vi "FilterChannels.vi"(8 "error in (no error)":errorcluster, 10 "Property":string, 11 "Specified Channel Ref List":T1[](array[typedef]) format="%.0x") -> (0 "error out":errorcluster, 3 "Filtered Channel list":T1[](array[typedef]) format="%.0x")   [LabVIEW 2020, in "Shared Variables CD 2.0 Engine.lvlib"]
doc: "Row 1: DBL\nRow 2 Bool"
uses:
  Shared Variables CD 2.0 Engine.lvlib
  <vilib>/NI VeriStand/Custom Device API/Custom Device Item Ref.ctl
  <vilib>/Utility/VariantDataType/Type.ctl
  <vilib>/Utility/VariantDataType/VariantType.lvlib
  <vilib>/NI VeriStand/Custom Device API/Custom Device API.lvlib
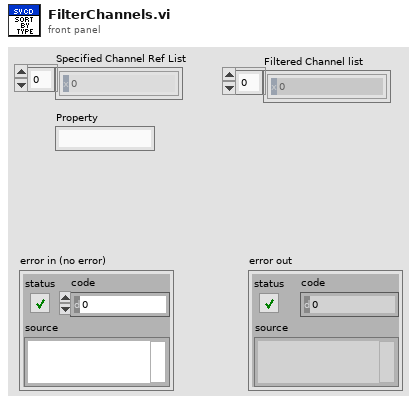
[diagram p1: front panel]
types:
  T1 = typedef "Custom Device API.lvlib/Custom Device Item Ref.ctl" = u64
  T2 = typedef "VariantType.lvlib/Type.ctl" = enum8{"Invalid Type", "Void", "I8", "I16", "I32", "I64", "U8", "U16", "U32", "U64", "Single Float", "Double Float", "Extended Float", "Single Complex", "Double Complex", "Extended Complex", "Enum U8", "Enum U16", "Enum U32", "Enum U64", "Single Float With Unit", "Double Float With Unit", "Extended Float With Unit", "Single Complex with Unit", "Double Complex with Unit", "Extended Complex with Unit", "Boolean", "String", "Path", "Picture", "Tag", "Array", "Cluster", "Variant", "LV Variant", "Waveform", "Timestamp", "Digital Waveform", "Digital Data", "ExpressData", "Refnum", "External Data", "VI", "Poly VI", "LabVIEW Class Instance", "Fixed Point"}
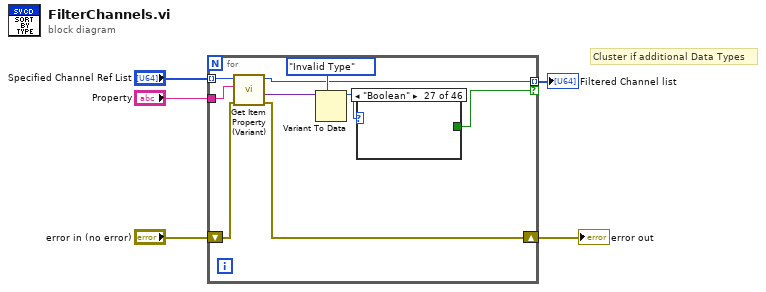
[diagram p0: block diagram]
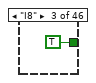
[diagram p4: hidden frame]
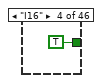
[diagram p5: hidden frame]
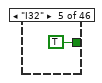
[diagram p6: hidden frame]
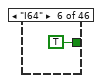
[diagram p7: hidden frame]
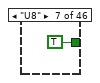
[diagram p8: hidden frame]
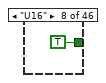
[diagram p9: hidden frame]
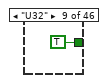
[diagram p10: hidden frame]
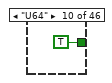
[diagram p11: hidden frame]
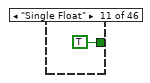
[diagram p12: hidden frame]
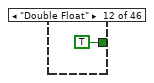
[diagram p13: hidden frame]
diagram:
  # "Cluster if additional Data Types"
  n1 = for {
    tunnel: "Specified Channel Ref List" -> [w10] mode=indexing
    tunnel: "Property" -> [w14]
    shift-right: [w8] -> w2
    shift-left: "error in (no error)" -> [w9]
    tunnel: [w7] -> w1 mode=indexing if=w6
    n2 = call <vilib>:"Get Item Property (Variant).vi"("error in (no error)"=w9, "Property Name"=w14, "Item Ref in"=w10) -> ("error out"=w8:errorcluster, "Value"=w13:variant, "Item Ref out"=w7:T1)  [unwired: 5 in, 1 out]
    n3 = Variant To Data(type=Type."Invalid Type" ("Type"), Variant=w13) -> (data=w11:T2)  [unwired: 1 in, 1 out]
    n4 = case shown="\"Boolean\"" w11 {
      tunnel: [_ _ TRUE TRUE TRUE TRUE TRUE TRUE TRUE TRUE TRUE TRUE _ _ _ _ _ _ _ _ _ _ _ _ _ _ _ _ _ _ _ _ _ _ _ _ _ _ _ _ _ _ _ _ _ _] -> w6
      frame "Invalid Type", Default {
      }
      frame "Void" {
      }
      frame "I8" {
      }
      frame "I16" {
      }
      frame "I32" {
      }
      frame "I64" {
      }
      frame "U8" {
      }
      frame "U16" {
      }
      frame "U32" {
      }
      frame "U64" {
      }
      frame "Single Float" {
      }
      frame "Double Float" {
      }
      frame "Extended Float" {
      }
      frame "Single Complex" {
      }
      frame "Double Complex" {
      }
      frame "Extended Complex" {
      }
      frame "Enum U8" {
      }
      frame "Enum U16" {
      }
      frame "Enum U32" {
      }
      frame "Enum U64" {
      }
      frame "Single Float With Unit" {
      }
      frame "Double Float With Unit" {
      }
      frame "Extended Float With Unit" {
      }
      frame "Single Complex with Unit" {
      }
      frame "Double Complex with Unit" {
      }
      frame "Extended Complex with Unit" {
      }
      frame "Boolean" {
      }
      frame "String" {
      }
      frame "Path" {
      }
      frame "Picture" {
      }
      frame "Tag" {
      }
      frame "Array" {
      }
      frame "Cluster" {
      }
      frame "Variant" {
      }
      frame "LV Variant" {
      }
      frame "Waveform" {
      }
      frame "Timestamp" {
      }
      frame "Digital Waveform" {
      }
      frame "Digital Data" {
      }
      frame "ExpressData" {
      }
      frame "Refnum" {
      }
      frame "External Data" {
      }
      frame "VI" {
      }
      frame "Poly VI" {
      }
      frame "LabVIEW Class Instance" {
      }
      frame "Fixed Point" {
      }
    }
  }
  "error out" <- w2
  "Filtered Channel list" <- w1
